vi "Istwert Ueberwachung.vi"(6 "Fehler Aktiviert?":bool=TRUE, 8 "Max":sgl, 9 "Min":sgl, 11 "Referernz":refnum<vi>) -> ()   [LabVIEW 2020, in "allgemeine Sub-VIs.lvlib"]
uses:
  allgemeine Sub-VIs.lvlib
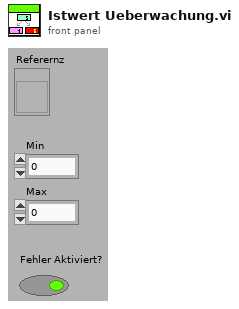
[diagram p1: front panel]
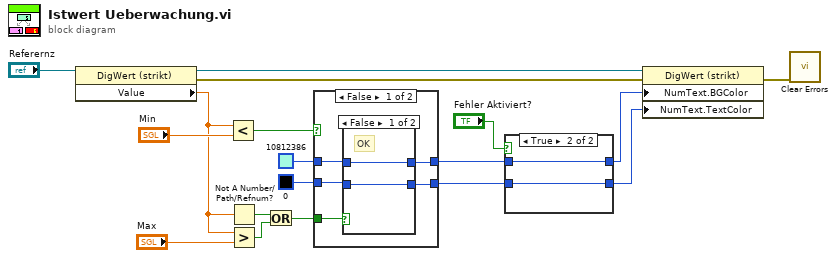
[diagram p0: block diagram]
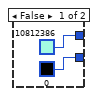
[diagram p2: hidden frame]
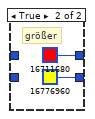
[diagram p3: hidden frame]
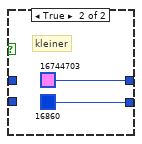
[diagram p4: hidden frame]
diagram:
  n1 = property class="DigWert (strikt)"(reference="Referernz") -> (reference out=w16:refnum<vi>, error out=w3:errorcluster, "Value"=w11:sgl)  [unwired: 1 in]
  n2 = Less?(x=w11, y="Min") -> (x < y?=w12:bool)
  n3 = Not A Number/Path/Refnum?(number/path/refnum=w11) -> (NaN/Path/Refnum?=w9:bool)
  n4 = Greater?(x=w11, y="Max") -> (0:w10:bool)
  n5 = Or(x=w9, y=w10) -> (x .or. y?=w1:bool)
  n6 = case shown="False" w12 {
    tunnel: u32 10812386 ("Hintergrund") -> [w23 _]
    tunnel: [w21 u32 16744703 ("Hintergrund")] -> w8
    tunnel: u32 0 ("Hintergrund") -> [w22 _]
    tunnel: [w20 u32 16860 ("Hintergrund")] -> w7
    tunnel: w1 -> [w19 _]
    frame False {
      n7 = case shown="False" w19 {
        tunnel: w23 -> [w25 _]
        tunnel: [w25 u32 16711680 ("Hintergrund")] -> w21
        tunnel: [w24 u32 16776960 ("Hintergrund")] -> w20
        tunnel: w22 -> [w24 _]
        frame False {
          # "OK"
        }
        frame True {
          # "größer"
        }
      }
    }
    frame True {
      # "kleiner"
    }
  }
  n8 = case shown="True" "Fehler Aktiviert?" {
    tunnel: w8 -> [_ w33]
    tunnel: w7 -> [_ w32]
    tunnel: [u32 10812386 ("Hintergrund") w33] -> w6
    tunnel: [u32 0 ("Hintergrund") w32] -> w5
    frame False {
    }
    frame True {
    }
  }
  n9 = property class="DigWert (strikt)"(reference=w16, error in=w3, "NumText.BGColor"=w6, "NumText.TextColor"=w5) -> (error out=w2:errorcluster)  [unwired: 1 out]
  n10 = call <vilib>:"Clear Errors.vi"("error in (no error)"=w2) -> ()  [unwired: 5 in, 2 out]
